vi "AGCxxx Revision Query.vi"(0 "AGCxxx VISA Cluster":T1={"VISA resource name"="", "VISA Timeout Value (1000 ms)"=1000, "Lock Timeout (1000 ms)"=1000, "MAX Channel (6)"=6}, 11 "error in (no error)":errorcluster) -> (4 "dup AGCxxx VISA Cluster":T1={"VISA resource name"="", "VISA Timeout Value (1000 ms)"=1000, "Lock Timeout (1000 ms)"=1000, "MAX Channel (6)"=6}, 8 "Instr Driver Revision":string, 10 "Instr Firmware Revision":string, 15 "error out":errorcluster)   [LabVIEW 2014, in "AGCxxx - Driver.lvlib"]
doc: "This VI queries the current instrument firmware revision and instrument driver revision.\n\nThis Instrument Driver's Revision number is XXX and is compatible with Instrument Firmware Revision XXX\n\n(Instrument Driver Name)\nCreated By: Kim Brueck\nRelease Date:\nOriginally Developed in LabVIEW Version: 6.0\n\nModification History: \n\nNone\n\n\nCopyright (C) \nGesellschaft f. Schwerionenforschung, GSI\nPlanckstr. 1\n64291 Darmstadt\nGermany\n\nContact: http://www-wnt.gsi.de/labview\n H.Brand@gsi.de\n\nThis program is free software; you can redistribute it and/or\nmodify it under the terms of the GNU General Public License\nas published by the Free Software Foundation; either version 2\nof the License, or (at your option) any later version.\n\nThis program is distributed in the hope that it will be useful,\nbut WITHOUT ANY WARRANTY; without even the implied warranty of\nMERCHANTABILITY or FITNESS FOR A PARTICULAR PURPOSE. See the\nGNU General Public License for more details (http://www.gnu.org)."
uses:
  AGCxxx - Driver.lvlib
  AGCxxx VISA Control.ctl
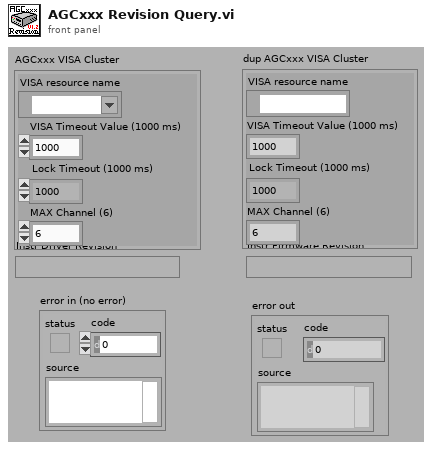
[diagram p1: front panel]
types:
  T1 = typedef "AGCxxx - Driver.lvlib/AGCxxx VISA Control.ctl" = cluster{"VISA resource name":refnum<visa-resource-name>, "VISA Timeout Value (1000 ms)":u32, "Lock Timeout (1000 ms)":u32, "MAX Channel (6)":i32}
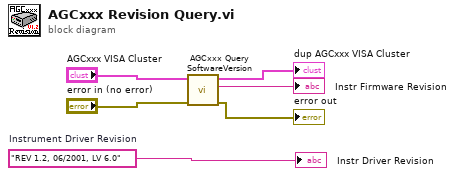
[diagram p0: block diagram]
diagram:
  w6 = "REV 1.2, 06/2001, LV 6.0"  # Instrument Driver Revision
  n1 = call "AGCxxx Query SoftwareVersion.vi"("error in (no error)"="error in (no error)", "AGCxxx VISA Cluster"="AGCxxx VISA Cluster") -> ("error out"=→"error out":errorcluster, "Version Number"=→"Instr Firmware Revision":string, "dup AGCxxx VISA Cluster"=→"dup AGCxxx VISA Cluster":T1)  [unwired: 6 in, 1 out]
  "Instr Driver Revision" <- w6
